vi "Load Becker-Hickl Measurement Stop Information.vi"(8 "error in (no error)":errorcluster, 10 "Measurement Stop Info in":T1 {"Flags" format="%.0b"}, 11 "string in":string) -> (0 "error out":errorcluster, 2 "Measurement Stop Info out":T1 {"Flags" format="%.0b"}, 3 "string out":string)   [LabVIEW 2021, in "Becker-Hickl Files.lvlib"]
uses:
  Becker-Hickl Files.lvlib
  Becker-Hickl Measurement Stop Info.ctl
  Becker-Hickl Read Single U16.vi
  Becker-Hickl Read Single SGL.vi
  Becker-Hickl Read Single I32.vi
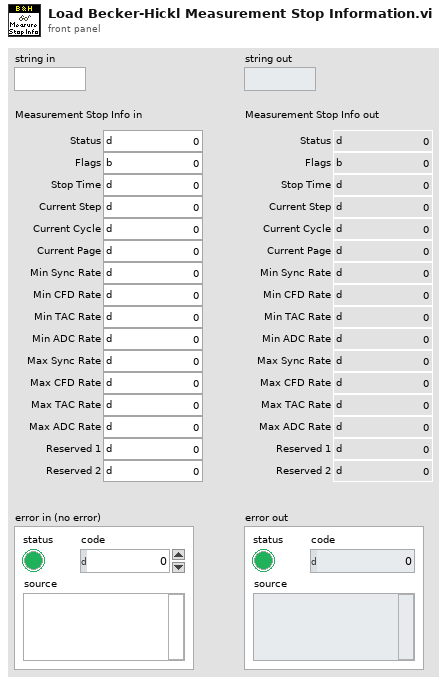
[diagram p1: front panel]
types:
  T1 = typedef "Becker-Hickl Files.lvlib/Becker-Hickl Measurement Stop Info.ctl" = cluster{"Status":u16, "Flags":u16, "Stop Time":sgl, "Current Step":i32, "Current Cycle":i32, "Current Page":i32, "Min Sync Rate":sgl, "Min CFD Rate":sgl, "Min TAC Rate":sgl, "Min ADC Rate":sgl, "Max Sync Rate":sgl, "Max CFD Rate":sgl, "Max TAC Rate":sgl, "Max ADC Rate":sgl, "Reserved 1":i32, "Reserved 2":sgl}
  T2 = enum16{"status", "flags", "stop_time", "cur_step", "cur_cycle", "cur_page", "min_sync_rate", "min_cfd_rate", "min_tac_rate", "min_adc_rate", "max_sync_rate", "max_cfd_rate", "max_tac_rate", "max_adc_rate", "reserved1", "reserved2"}
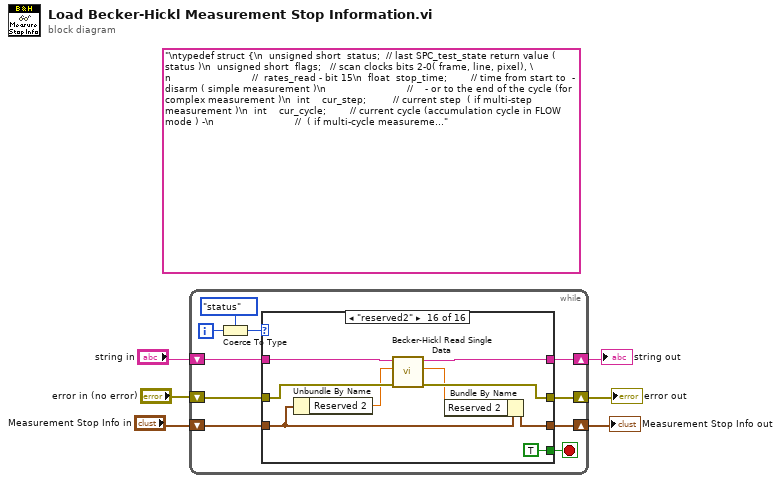
[diagram p0: block diagram]
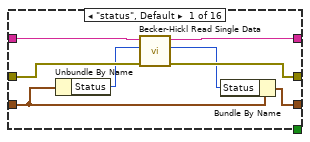
[diagram p2: hidden frame]
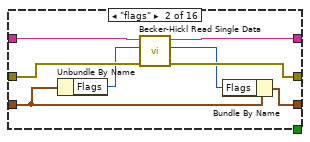
[diagram p3: hidden frame]
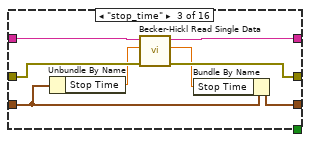
[diagram p4: hidden frame]
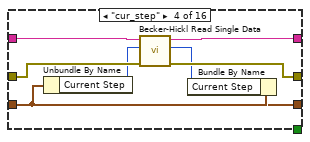
[diagram p5: hidden frame]
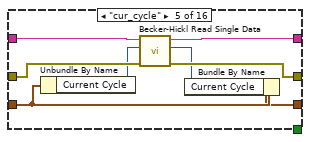
[diagram p6: hidden frame]
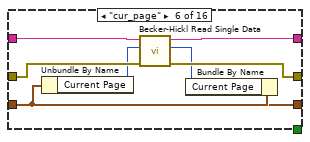
[diagram p7: hidden frame]
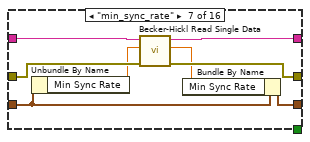
[diagram p8: hidden frame]
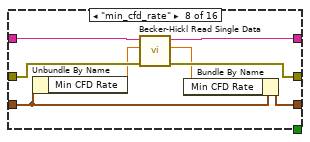
[diagram p9: hidden frame]
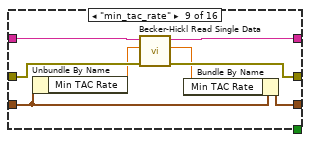
[diagram p10: hidden frame]
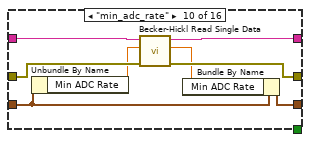
[diagram p11: hidden frame]
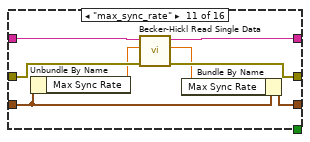
[diagram p12: hidden frame]
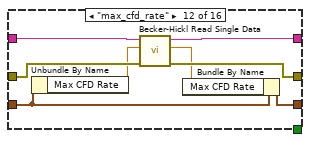
[diagram p13: hidden frame]
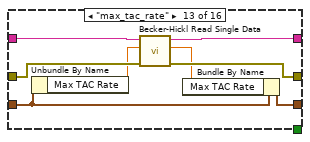
[diagram p14: hidden frame]
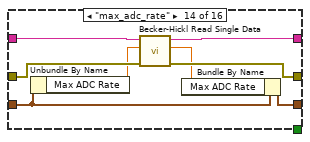
[diagram p15: hidden frame]
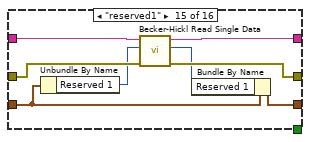
[diagram p16: hidden frame]
diagram:
  (unwired) "\ntypedef struct {\n  unsigned short  status;  // last SPC_test_state return value ( status )\n  unsigned short  flags;   // scan clocks bits 2-0( frame, line, pixel), \n                           //  rates_read - bit 15\n  float  stop_time;        // time from start to  - disarm ( simple measurement )\n                           //    - or to the end of the cycle (for complex measurement )\n  int    cur_step;         // current step  ( if multi-step measurement )\n  int    cur_cycle;        // current cycle (accumulation cycle in FLOW mode ) -\n                           //  ( if multi-cycle measurement ) \n  int    cur_page;         // current measured page\n  float  min_sync_rate;    // minimum rates during the measurement\n  float  min_cfd_rate;     //   ( -1.0 - not set )\n  float  min_tac_rate;\n  float  min_adc_rate;\n  float  max_sync_rate;    // maximum rates during the measurement\n  float  max_cfd_rate;     //   ( -1.0 - not set )\n  float  max_tac_rate;\n  float  max_adc_rate;\n  int    reserved1;\n  float  reserved2;\n  }MeasStopInfo;           // information collected when measurement is finished\n "
  n1 = while {
    shift-right: [w9] -> w1
    shift-left: "string in" -> [w10]
    shift-right: [w11] -> w2
    shift-left: "error in (no error)" -> [w12]
    shift-right: [w13] -> w3
    shift-left: "Measurement Stop Info in" -> [w14]
    i -> [w16]
    stop <- w7 stop-if-true
    n2 = Coerce To Type(0:w16, 1:T2."status") -> (2:w15:T2)
    n3 = case shown="\"reserved2\"" w15 {
      tunnel: w14 -> [w20 w28 w36 w44 w52 w60 w68 w76 w84 w92 w100 w108 w116 w124 w132 w141]
      tunnel: [w18 w26 w34 w42 w50 w58 w66 w74 w82 w90 w98 w106 w114 w122 w130 w139] -> w13
      tunnel: w12 -> [w21 w29 w37 w45 w53 w61 w69 w77 w85 w93 w101 w109 w117 w125 w133 w142]
      tunnel: [w22 w30 w38 w46 w54 w62 w70 w78 w86 w94 w102 w110 w118 w126 w134 w143] -> w11
      tunnel: w10 -> [w24 w32 w40 w48 w56 w64 w72 w80 w88 w96 w104 w112 w120 w128 w136 w145]
      tunnel: [w23 w31 w39 w47 w55 w63 w71 w79 w87 w95 w103 w111 w119 w127 w135 w144] -> w9
      tunnel: [_ _ _ _ _ _ _ _ _ _ _ _ _ _ _ TRUE] -> w7
      frame "status", Default {
        n4 = Unbundle By Name(w20) -> ("Status"=w19:u16)
        n5 = call-poly "Becker-Hickl Read Single Data.vi"("Error In"=w21, "Default"=w19, "Bytes in"=w24) -> ("Error Out"=w22:errorcluster, "U16"=w17:u16, "Bytes out"=w23:string)  [unwired: 6 in]
        n6 = Bundle By Name(cluster=w20, "Status"=w17) -> (w18:T1)
      }
      frame "flags" {
        n7 = Unbundle By Name(w28) -> ("Flags"=w27:u16)
        n8 = call-poly "Becker-Hickl Read Single Data.vi"("Error In"=w29, "Default"=w27, "Bytes in"=w32) -> ("Error Out"=w30:errorcluster, "U16"=w25:u16, "Bytes out"=w31:string)  [unwired: 6 in]
        n9 = Bundle By Name(cluster=w28, "Flags"=w25) -> (w26:T1)
      }
      frame "stop_time" {
        n10 = Unbundle By Name(w36) -> ("Stop Time"=w35:sgl)
        n11 = call-poly "Becker-Hickl Read Single Data.vi"("Error In"=w37, "Default"=w35, "Bytes in"=w40) -> ("Error Out"=w38:errorcluster, "SGL"=w33:sgl, "Bytes out"=w39:string)  [unwired: 6 in]
        n12 = Bundle By Name(cluster=w36, "Stop Time"=w33) -> (w34:T1)
      }
      frame "cur_step" {
        n13 = Unbundle By Name(w44) -> ("Current Step"=w43:i32)
        n14 = call-poly "Becker-Hickl Read Single Data.vi"("Error In"=w45, "Default"=w43, "Bytes in"=w48) -> ("Error Out"=w46:errorcluster, "I32"=w41:i32, "Bytes out"=w47:string)  [unwired: 6 in]
        n15 = Bundle By Name(cluster=w44, "Current Step"=w41) -> (w42:T1)
      }
      frame "cur_cycle" {
        n16 = Unbundle By Name(w52) -> ("Current Cycle"=w51:i32)
        n17 = call-poly "Becker-Hickl Read Single Data.vi"("Error In"=w53, "Default"=w51, "Bytes in"=w56) -> ("Error Out"=w54:errorcluster, "I32"=w49:i32, "Bytes out"=w55:string)  [unwired: 6 in]
        n18 = Bundle By Name(cluster=w52, "Current Cycle"=w49) -> (w50:T1)
      }
      frame "cur_page" {
        n19 = Unbundle By Name(w60) -> ("Current Page"=w59:i32)
        n20 = call-poly "Becker-Hickl Read Single Data.vi"("Error In"=w61, "Default"=w59, "Bytes in"=w64) -> ("Error Out"=w62:errorcluster, "I32"=w57:i32, "Bytes out"=w63:string)  [unwired: 6 in]
        n21 = Bundle By Name(cluster=w60, "Current Page"=w57) -> (w58:T1)
      }
      frame "min_sync_rate" {
        n22 = Unbundle By Name(w68) -> ("Min Sync Rate"=w67:sgl)
        n23 = call-poly "Becker-Hickl Read Single Data.vi"("Error In"=w69, "Default"=w67, "Bytes in"=w72) -> ("Error Out"=w70:errorcluster, "SGL"=w65:sgl, "Bytes out"=w71:string)  [unwired: 6 in]
        n24 = Bundle By Name(cluster=w68, "Min Sync Rate"=w65) -> (w66:T1)
      }
      frame "min_cfd_rate" {
        n25 = Unbundle By Name(w76) -> ("Min CFD Rate"=w75:sgl)
        n26 = call-poly "Becker-Hickl Read Single Data.vi"("Error In"=w77, "Default"=w75, "Bytes in"=w80) -> ("Error Out"=w78:errorcluster, "SGL"=w73:sgl, "Bytes out"=w79:string)  [unwired: 6 in]
        n27 = Bundle By Name(cluster=w76, "Min CFD Rate"=w73) -> (w74:T1)
      }
      frame "min_tac_rate" {
        n28 = Unbundle By Name(w84) -> ("Min TAC Rate"=w83:sgl)
        n29 = call-poly "Becker-Hickl Read Single Data.vi"("Error In"=w85, "Default"=w83, "Bytes in"=w88) -> ("Error Out"=w86:errorcluster, "SGL"=w81:sgl, "Bytes out"=w87:string)  [unwired: 6 in]
        n30 = Bundle By Name(cluster=w84, "Min TAC Rate"=w81) -> (w82:T1)
      }
      frame "min_adc_rate" {
        n31 = Unbundle By Name(w92) -> ("Min ADC Rate"=w91:sgl)
        n32 = call-poly "Becker-Hickl Read Single Data.vi"("Error In"=w93, "Default"=w91, "Bytes in"=w96) -> ("Error Out"=w94:errorcluster, "SGL"=w89:sgl, "Bytes out"=w95:string)  [unwired: 6 in]
        n33 = Bundle By Name(cluster=w92, "Min ADC Rate"=w89) -> (w90:T1)
      }
      frame "max_sync_rate" {
        n34 = Unbundle By Name(w100) -> ("Max Sync Rate"=w99:sgl)
        n35 = call-poly "Becker-Hickl Read Single Data.vi"("Error In"=w101, "Default"=w99, "Bytes in"=w104) -> ("Error Out"=w102:errorcluster, "SGL"=w97:sgl, "Bytes out"=w103:string)  [unwired: 6 in]
        n36 = Bundle By Name(cluster=w100, "Max Sync Rate"=w97) -> (w98:T1)
      }
      frame "max_cfd_rate" {
        n37 = Unbundle By Name(w108) -> ("Max CFD Rate"=w107:sgl)
        n38 = call-poly "Becker-Hickl Read Single Data.vi"("Error In"=w109, "Default"=w107, "Bytes in"=w112) -> ("Error Out"=w110:errorcluster, "SGL"=w105:sgl, "Bytes out"=w111:string)  [unwired: 6 in]
        n39 = Bundle By Name(cluster=w108, "Max CFD Rate"=w105) -> (w106:T1)
      }
      frame "max_tac_rate" {
        n40 = Unbundle By Name(w116) -> ("Max TAC Rate"=w115:sgl)
        n41 = call-poly "Becker-Hickl Read Single Data.vi"("Error In"=w117, "Default"=w115, "Bytes in"=w120) -> ("Error Out"=w118:errorcluster, "SGL"=w113:sgl, "Bytes out"=w119:string)  [unwired: 6 in]
        n42 = Bundle By Name(cluster=w116, "Max TAC Rate"=w113) -> (w114:T1)
      }
      frame "max_adc_rate" {
        n43 = Unbundle By Name(w124) -> ("Max ADC Rate"=w123:sgl)
        n44 = call-poly "Becker-Hickl Read Single Data.vi"("Error In"=w125, "Default"=w123, "Bytes in"=w128) -> ("Error Out"=w126:errorcluster, "SGL"=w121:sgl, "Bytes out"=w127:string)  [unwired: 6 in]
        n45 = Bundle By Name(cluster=w124, "Max ADC Rate"=w121) -> (w122:T1)
      }
      frame "reserved1" {
        n46 = Unbundle By Name(w132) -> ("Reserved 1"=w131:i32)
        n47 = call-poly "Becker-Hickl Read Single Data.vi"("Error In"=w133, "Default"=w131, "Bytes in"=w136) -> ("Error Out"=w134:errorcluster, "I32"=w129:i32, "Bytes out"=w135:string)  [unwired: 6 in]
        n48 = Bundle By Name(cluster=w132, "Reserved 1"=w129) -> (w130:T1)
      }
      frame "reserved2" {
        n49 = Unbundle By Name(w141) -> ("Reserved 2"=w140:sgl)
        n50 = call-poly "Becker-Hickl Read Single Data.vi"("Error In"=w142, "Default"=w140, "Bytes in"=w145) -> ("Error Out"=w143:errorcluster, "SGL"=w138:sgl, "Bytes out"=w144:string)  [unwired: 6 in]
        n51 = Bundle By Name(cluster=w141, "Reserved 2"=w138) -> (w139:T1)
      }
    }
  }
  "Measurement Stop Info out" <- w3
  "error out" <- w2
  "string out" <- w1
